vi "Module Loop.vi"(8 "error in (no error)":errorcluster, 11 "Historian Module in":refnum<class "Historian Module.lvclass">) -> (0 "error out":errorcluster, 3 "Historian Module out":refnum<class "Historian Module.lvclass">)   [LabVIEW 2020, in "VolatusHistorian.lvlib" / "Historian Module.lvclass"]
uses:
  Historian Module.lvclass
  C:/dev/lv20CE/relink/lv-volatus/Volatus/Module/Module.lvclass
  Volatus/Module/Module.lvclass
  Data Request.ctl
  Time Format.ctl
  Volatus/MessageQ/MessageQ.lvclass
  Volatus/MessageQ/MessageQ.lvclass/MessageQ.ctl
  Historian Module.lvclass/Historian Module.ctl
  Volatus/Module/Module.lvclass/Module.ctl
  lv-promises/Promises/Promise/Promise.lvclass
  C:/dev/lv20CE/relink/lv-volatus/VolatusHistorian/Historian Module/Historian Module.lvclass
  VolatusHistorian.lvlib
  Group Buffer DBL/Group Buffer DBL.lvclass
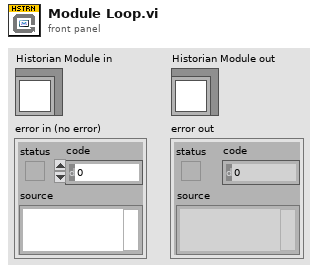
[diagram p1: front panel]
types:
  T1 = enum32{"Invalid", "Standard", "Closed", "Hidden", "Minimized", "Maximized"}
  T2 = typedef "VolatusHistorian.lvlib/Data Request.ctl" = cluster{"Channels":string[], "Start Time":dbl, "End Time":dbl, "Time Format":T3}
  T3 = typedef "VolatusHistorian.lvlib/Time Format.ctl" = enum16{"unix_ns", "lv"}
  T4 = map{string, refnum<class "Group Buffer DBL.lvclass">}
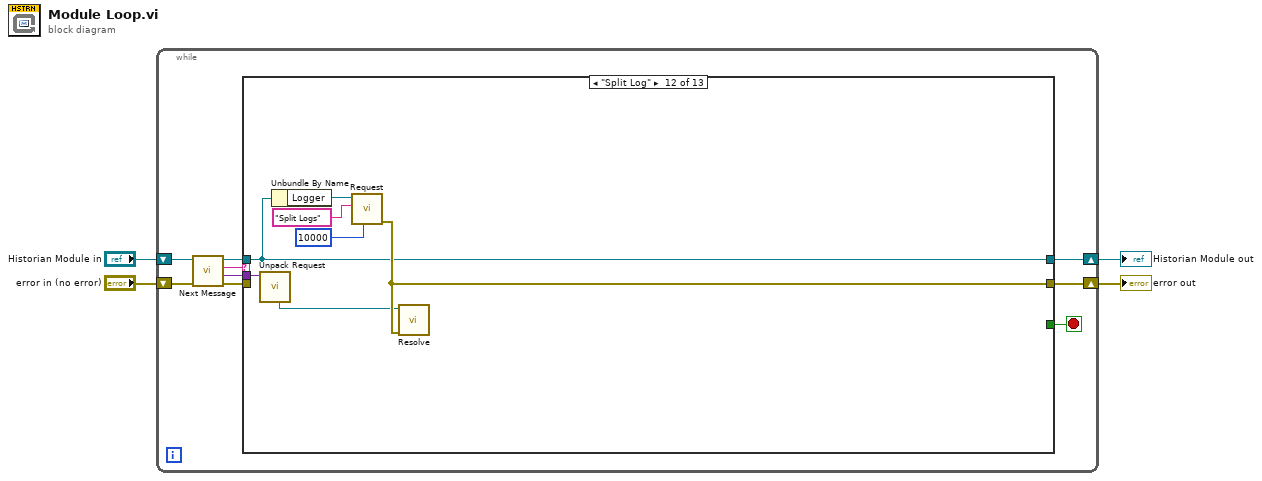
[diagram p0: block diagram]
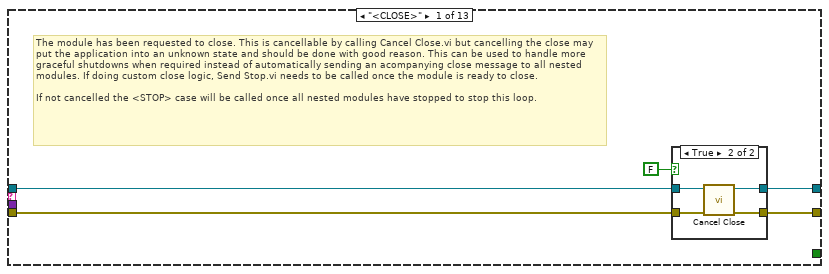
[diagram p2: hidden frame]
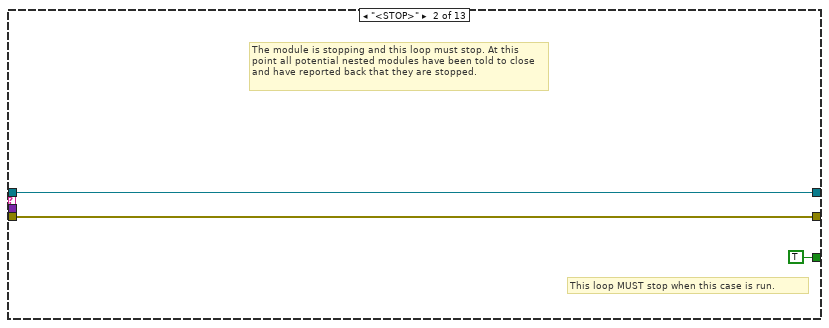
[diagram p4: hidden frame]
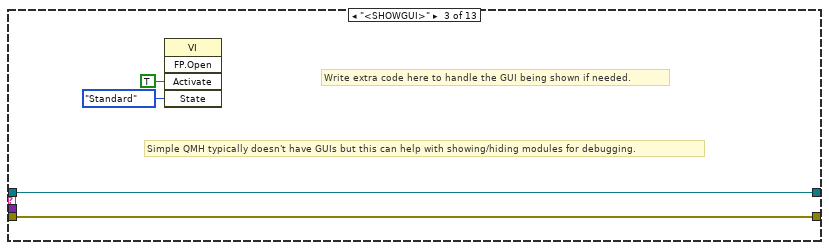
[diagram p5: hidden frame]
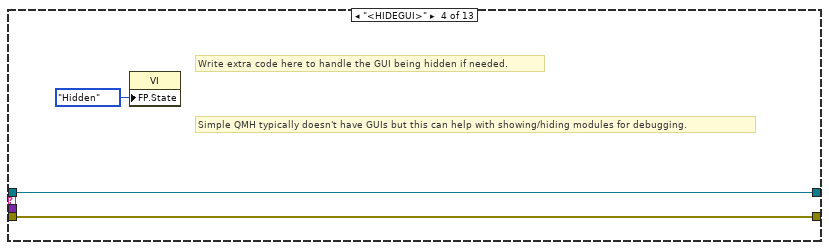
[diagram p6: hidden frame]
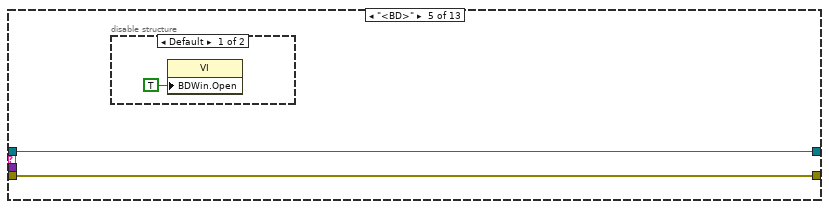
[diagram p7: hidden frame]
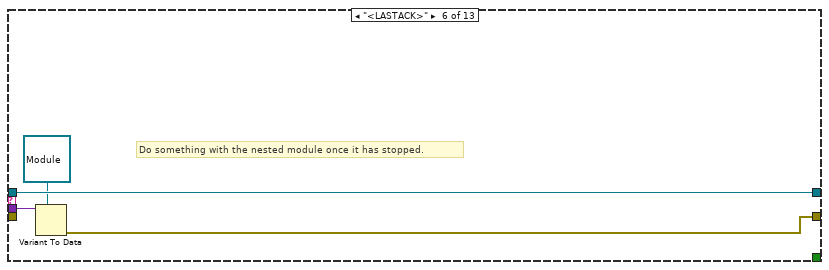
[diagram p9: hidden frame]
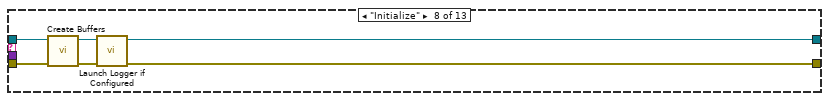
[diagram p11: hidden frame]
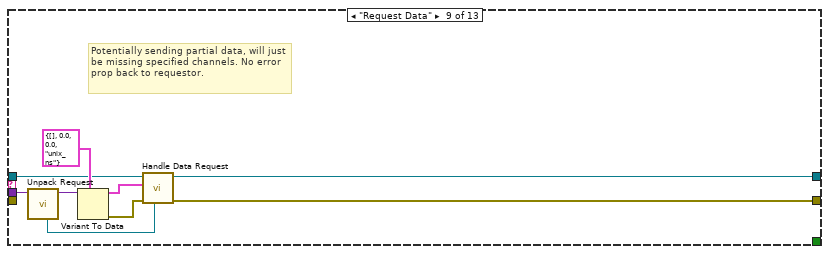
[diagram p12: hidden frame]
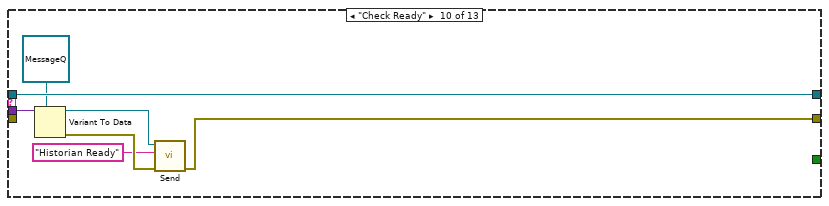
[diagram p13: hidden frame]
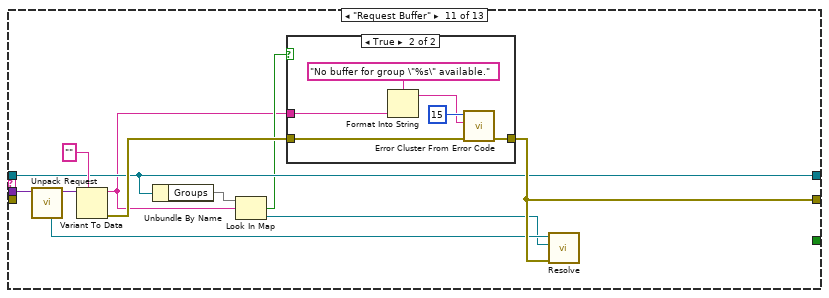
[diagram p14: hidden frame]
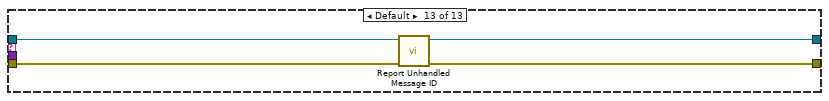
[diagram p16: hidden frame]
diagram:
  n1 = while {
    shift-right: [w8] -> w1
    shift-left: "Historian Module in" -> [w13]
    shift-right: [w5] -> w2
    shift-left: "error in (no error)" -> [w12]
    stop <- w7 stop-if-true
    n2 = call "Next Message.vi"("error in (no error)"=w12, "Module in"=w13) -> ("error out"=w11:errorcluster, "Data"=w6:variant, "ID"=w10:string, "Module out"=w9:refnum<class "Historian Module.lvclass">)  [unwired: 6 in]
    n3 = case shown="\"Split Log\"" w10 {
      tunnel: w11 -> [w18 w26 w30 w33 w35 _ w42 w49 _ _ _ _ w94]
      tunnel: w9 -> [w16 w27 w31 w34 w36 w41 w43 w47 w55 w64 w70 w89 w92]
      tunnel: [w15 w27 w31 w34 w36 w41 w43 w44 w54 w64 w70 w89 w91] -> w8
      tunnel: [_ TRUE _ _ _ _ _ _ _ _ _ _ _] -> w7
      tunnel: w6 -> [_ _ _ _ _ w40 _ _ w58 w63 w74 w88 _]
      tunnel: [w17 w26 w30 w33 w35 w38 w42 w46 w50 w59 w76 w90 w93] -> w5
      frame "<CLOSE>" {
        # "The module has been requested to close. This is cancellable by calling Cancel Close.vi but cancelling the close may put the application into an unknown state and should be done with good reason. This can be used to handle more graceful shutdowns when required instead of automatically sending an acompanying close message to all nested modules. If doing custom close logic, Send Stop.vi needs to be called once the module is ready to close.\n\nIf not cancelled the <STOP> case will be called once all nested modules have stopped to stop this loop."
        n4 = case shown="True" FALSE {
          tunnel: w18 -> [w19 w24]
          tunnel: [w19 w23] -> w17
          tunnel: w16 -> [w20 w22]
          tunnel: [w20 w21] -> w15
          frame False {
          }
          frame True {
            n5 = call "Cancel Close.vi"("error in (no error)"=w24, "Module in"=w22) -> ("error out"=w23:errorcluster, "Module out"=w21:refnum<class "Historian Module.lvclass">)  [unwired: 8 in]
          }
        }
      }
      frame "<STOP>" {
        # "This loop MUST stop when this case is run."
        # "The module is stopping and this loop must stop. At this point all potential nested modules have been told to close and have reported back that they are stopped."
      }
      frame "<SHOWGUI>" {
        # "Simple QMH typically doesn't have GUIs but this can help with showing/hiding modules for debugging."
        # "Write extra code here to handle the GUI being shown if needed."
        n6 = invoke class="VI" method="FP.Open"("Activate"=TRUE ("Activate?"), "State"=T1."Standard") -> ()  [unwired: 3 in, 5 out]
      }
      frame "<HIDEGUI>" {
        # "Simple QMH typically doesn't have GUIs but this can help with showing/hiding modules for debugging."
        # "Write extra code here to handle the GUI being hidden if needed."
        n7 = property class="VI"("FP.State"=T1."Hidden" ("Front Panel Window:State")) -> ()  [unwired: 2 in, 2 out]
      }
      frame "<BD>" {
        n8 = disable-structure shown="Default" {
          frame condition #0 (active) {
            n9 = property class="VI"("BDWin.Open"=TRUE ("Block Diagram Window:Open")) -> ()  [unwired: 2 in, 2 out]
          }
          frame condition #1 {
          }
        }
      }
      frame "<LASTACK>" {
        # "Do something with the nested module once it has stopped."
        n10 = Variant To Data(type=refnum<class "Module.lvclass"> refnum ("Volatus:Module"), Variant=w40) -> (error out=w38:errorcluster)  [unwired: 1 in, 1 out]
      }
      frame "<TIMEOUT>" {
        # "No message for this module was received in time"
      }
      frame "Initialize" {
        n11 = call "Create Buffers.vi"("error in (no error)"=w49, "Historian Module in"=w47) -> ("error out"=w48:errorcluster, "Historian Module out"=w45:refnum<class "Historian Module.lvclass">)  [unwired: 8 in]
        n12 = call "Launch Logger if Configured.vi"("error in (no error)"=w48, "Historian Module in"=w45) -> ("error out"=w46:errorcluster, "Historian Module out"=w44:refnum<class "Historian Module.lvclass">)  [unwired: 8 in]
      }
      frame "Request Data" {
        # "Potentially sending partial data, will just be missing specified channels. No error prop back to requestor."
        n13 = call "Unpack Request.vi"("Request Data"=w58) -> ("Data"=w57:variant, "Promise"=w52:refnum<class "Promise.lvclass">)  [unwired: 8 in, 1 out]
        n14 = Variant To Data(type=T2 {"Channels"=[], "Start Time"=0.0, "End Time"=0.0, "Time Format"=enum."unix_ns"} ("Data Request"), Variant=w57) -> (data=w53:T2, error out=w51:errorcluster)  [unwired: 1 in]
        n15 = call "Handle Data Request.vi"("Promise"=w52, "error in (no error)"=w51, "Data Request"=w53, "Historian Module in"=w55) -> ("error out"=w50:errorcluster, "Historian Module out"=w54:refnum<class "Historian Module.lvclass">)  [unwired: 6 in]
      }
      frame "Check Ready" {
        n16 = Variant To Data(type=refnum<class "MessageQ.lvclass"> refnum ("Volatus:MessageQ"), Variant=w63) -> (data=w61:refnum<class "MessageQ.lvclass">, error out=w65:errorcluster)  [unwired: 1 in]
        n17 = call "Send.vi"("error in (no error)"=w65, "ID"="Historian Ready", "MessageQ in"=w61) -> ("error out"=w59:errorcluster)  [unwired: 7 in, 1 out]
      }
      frame "Request Buffer" {
        n18 = call "Unpack Request.vi"("Request Data"=w74) -> ("Data"=w72:variant, "Promise"=w73:refnum<class "Promise.lvclass">)  [unwired: 8 in, 1 out]
        n19 = Variant To Data(type="", Variant=w72) -> (data=w66:string, error out=w75:errorcluster)  [unwired: 1 in]
        n20 = Unbundle By Name(w70) -> ("Groups"=w69:T4)
        n21 = Look In Map(map=w69, key=w66) -> (key not found?=w67:bool, value=w68:refnum<class "Group Buffer DBL.lvclass">)  [unwired: 1 in]
        n22 = case shown="True" w67 {
          tunnel: w66 -> [_ w80]
          tunnel: [w77 w79] -> w76
          tunnel: w75 -> [w77 w78]
          frame False {
          }
          frame True {
            n23 = Format Into String(format string="No buffer for group \"%s\" available.", w80) -> (resulting string=w81:string)  [unwired: 2 in, 1 out]
            n24 = call <vilib>:"Error Cluster From Error Code.vi"("error in (no error)"=w78, "error message (\"\")"=w81, "error code (0)"=15) -> ("error out"=w79:errorcluster)  [unwired: 6 in]
          }
        }
        n25 = call "Resolve.vi"("error in (no error)"=w76, "Result (None)"=w68, "Promise in"=w73) -> ()  [unwired: 7 in, 2 out]
      }
      frame "Split Log" {
        n26 = call "Unpack Request.vi"("Request Data"=w88) -> ("Promise"=w85:refnum<class "Promise.lvclass">)  [unwired: 8 in, 2 out]
        n27 = Unbundle By Name(w89) -> ("Logger"=w87:refnum<class "MessageQ.lvclass">)
        n28 = call "Request.vi"("Timeout ms (1000)"=10000, "ID"="Split Logs", "MessageQ in"=w87) -> ("error out"=w90:errorcluster)  [unwired: 6 in, 2 out]
        n29 = call "Resolve.vi"("error in (no error)"=w90, "Promise in"=w85) -> ()  [unwired: 8 in, 2 out]
      }
      frame Default {
        n30 = call "Report Unhandled Message ID.vi"("error in (no error)"=w94, "Module in"=w92) -> ("error out"=w93:errorcluster, "Module out"=w91:refnum<class "Historian Module.lvclass">)  [unwired: 8 in]
      }
    }
  }
  "error out" <- w2
  "Historian Module out" <- w1
